vi "Waveform Replication (FPGA).vi"() -> ()   [LabVIEW 2019]
doc: "This VI is the controlling VI running on an FPGA target. This VI implements the closed-loop control algorithm based on an LMS adaptive filter. This VI acquires the actual vibration of the shaker, regulates the driving signal for the shaker, and builds the inverse model of the shaker with an LMS filter. The FXP LMS VI implements the LMS adaptive filter algorithm. Use the IP Generator to generate the FXP LMS VI. After you modify this VI or if you want to use this VI on a different CompactRIO chassis, you need to re-compile this VI."
uses:
  <vilib>/LabVIEW Targets/FPGA/cRIO/shared/nicrio_ModuleControls/nicrio_cRIO-9233_DataRatesRing.ctl
  <vilib>/rvi/eio/common/nirviEmuTemplateMethod_errors.vi
  <vilib>/rvi/eio/common/nirviEmuTemplatePropertySet_noerrors.vi
  <vilib>/rvi/Emulation/niFpgaGetClockAttributes.vi
  <vilib>/rvi/Emulation/niFpgaSctlEmulationGetInTimedLoop.vi
  <vilib>/rvi/Emulation/niFpgaEmulationReportErrorSimple.vi
  <vilib>/rvi/interface/RandomDataEmulation/niFpgaRandomDataHandleErrors.vi
  <vilib>/rvi/Emulation/niFpgaCriticalErrorInLSC.vi
  <vilib>/eio/EIONode/EIONode.xnode
  <vilib>/eio/EIOPropertyNode/EIOPropertyNode.xnode
  <vilib>/LabVIEW Targets/FPGA/cRIO/shared/nicrio_ModuleControls/nicrio_cRIO-9234_DataRatesRing2.ctl
  <vilib>/rvi/DataTransferAndStorage/Container/XNode/niFpgaContainer.xnode
  <vilib>/rvi/interface/RandomDataEmulation/nirviRandomDataFpgaReadWriteTemplate.vi
  <vilib>/rvi/eio/common/nirviEmuTemplatePropertyGet_errors.vi
  <vilib>/rvi/eio/common/nirviEmuTemplatePropertyGet_noerrors.vi
  <vilib>/rvi/eio/common/nirviEmuTemplatePropertySet_errors.vi
panel:
  in  "delay":i16=500
  in  "reset? (F)":bool
  out "e(n)":fxp<+/-,24,4> format="%.22g"
  in  "step size":fxp<+/-,16,-1>
  in  "control on?":bool
  in  "stop":bool
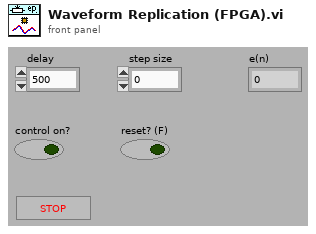
[diagram p1: front panel]
types:
  T1 = typedef "nicrio_cRIO-9233_DataRatesRing.ctl" = u8
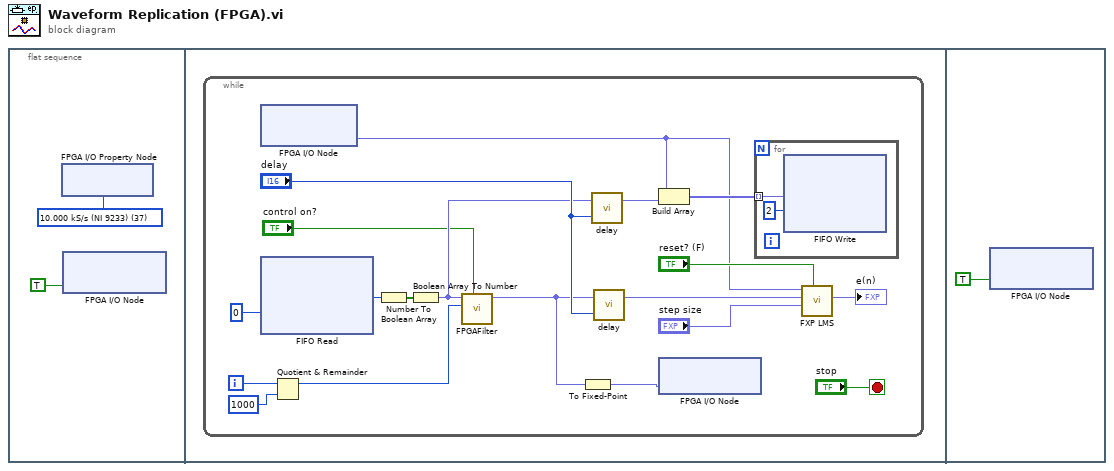
[diagram p0: block diagram]
diagram:
  n1 = flat-sequence {
    frame #0 {
      w1 = T1 37 items=["50.000 kS/s (NI 9233)"=2, "33.333 kS/s (NI 9233)"=3, "25.000 kS/s (NI 9233)"=34, "16.667 kS/s (NI 9233)"=35, "12.500 kS/s (NI 9233)"=36, "10.000 kS/s (NI 9233)"=37, "  8.333 kS/s (NI 9233)"=38, "  7.143 kS/s (NI 9233)"=39, "  6.250 kS/s (NI 9233)"=40, "  5.556 kS/s (NI 9233)"=41, "  5.000 kS/s (NI 9233)"=42, "  4.545 kS/s (NI 9233)"=43, "  4.167 kS/s (NI 9233)"=44, "  3.846 kS/s (NI 9233)"=45, "  3.571 kS/s (NI 9233)"=46, "  3.333 kS/s (NI 9233)"=47, "  3.125 kS/s (NI 9233)"=48, "  2.941 kS/s (NI 9233)"=49, "  2.778 kS/s (NI 9233)"=50, "  2.632 kS/s (NI 9233)"=51, "  2.500 kS/s (NI 9233)"=52, "  2.381 kS/s (NI 9233)"=53, "  2.273 kS/s (NI 9233)"=54, "  2.174 kS/s (NI 9233)"=55, "  2.083 kS/s (NI 9233)"=56, "  2.000 kS/s (NI 9233)"=57] ("Data Rate")
      n2 = xnode "FPGA I/O Property Node"("Data Rate"=w1) -> ()  [unwired: 1 in, 1 out]
      n3 = xnode "FPGA I/O Node"("Mod1/Start"=TRUE) -> ()  [unwired: 2 in, 2 out]
    }
    frame #1 {
      n4 = while {
        i -> [w6]
        stop <- "stop" stop-if-true
        n5 = xnode "FPGA I/O Node"() -> ("Mod1/AI0"=w13:fxp<+/-,24,4>)  [unwired: 2 in, 2 out]
        n6 = xnode ("FIFO Read")("Timeout"=0) -> ("Element"=w9:i32)  [unwired: 1 in, 2 out]
        n7 = Quotient & Remainder(x=w6, y=1000) -> (x-y*floor(x/y)=w3:i32)  [unwired: 1 out]
        n8 = Number To Boolean Array(number=w9) -> (Boolean array=w8:bool[])
        n9 = Boolean Array To Number(Boolean array=w8) -> (number=w7:fxp<+/-,24,4>)
        n10 = call "FPGAFilter.vi"("filter on"="control on?", "coeff addr"=w3, "x"=w7) -> ("y"=w12:fxp<+/-,24,4>)  [unwired: 1 in, 7 out]
        n11 = To Fixed-Point(number=w12) -> (fixed-point=w11:fxp<+/-,20,5>)  [unwired: 1 out]
        n12 = call "delay.vi"("delay"="delay", "x(n)"=w7) -> ("x(n-N)"=w18:fxp<+/-,24,4>)  [unwired: 1 out]
        n13 = call "delay.vi"("delay"="delay", "x(n)"=w12) -> ("x(n-N)"=w10:fxp<+/-,24,4>)  [unwired: 1 out]
        n14 = Build Array(w13, w18) -> (w19:fxp<+/-,24,4>[])
        n15 = xnode "FPGA I/O Node"("Mod2/AO0"=w11) -> ()  [unwired: 1 in, 1 out]
        n16 = for {
          tunnel: w19 -> [w22] mode=indexing
          n17 = xnode ("FIFO Write")("Element"=w22, "Timeout"=2) -> ()  [unwired: 1 in, 2 out]
        }
        n18 = call "FXP LMS.vi"("reset? (F)"="reset? (F)", "step size"="step size", "d(n)"=w10, "x(n)"=w13) -> ("e(n)"=→"e(n)":fxp<+/-,24,4>)  [unwired: 1 in, 6 out]
      }
    }
    frame #2 {
      n19 = xnode "FPGA I/O Node"("Mod1/Stop"=TRUE) -> ()  [unwired: 2 in, 2 out]
    }
  }
